vi "APS start sscnet.vi"(8 "error in (no error)":errorcluster caption="错误输入（无错误）", 10 "AxisFound_InBits":i32, 11 "Board_ID":i32) -> (0 "error out":errorcluster caption="错误输出", 2 "AxisFound_InBits out":i32, 3 "function return":i32)   [LabVIEW 2011, in "APS168.lvlib"]
doc: "I32 FNTYPE APS_start_sscnet( I32 Board_ID, I32 *AxisFound_InBits );"
uses:
  APS168.lvlib
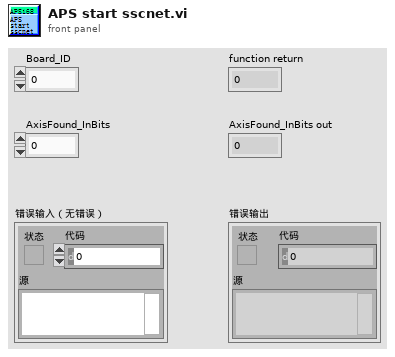
[diagram p1: front panel]
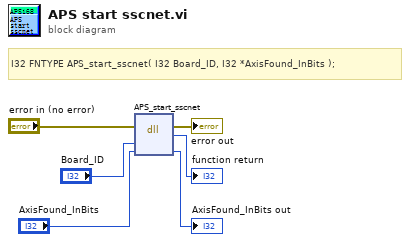
[diagram p0: block diagram]
diagram:
  # "I32 FNTYPE APS_start_sscnet( I32 Board_ID, I32 *AxisFound_InBits );"
  n1 = dll-call lib="PTH1Labs E软件ADLINK 204CAPS_1_7_1_LIB line 连续运动204APS168.*" fn="APS_start_sscnet"(error in="error in (no error)", "Board_ID"="Board_ID", "AxisFound_InBits"="AxisFound_InBits") -> (error out=→"error out":errorcluster, →"function return":i32, "AxisFound_InBits"=→"AxisFound_InBits out":i32)  [unwired: 3 in, 1 out]
